vi "Get_Variant_Cluster_Element_Names.vi"(8 "error in (no error)":errorcluster, 11 "Cluster in":variant) -> (0 "error out":errorcluster, 2 "Element names":string[](array[string]), 3 "Cluster out":variant)   [LabVIEW 2012]
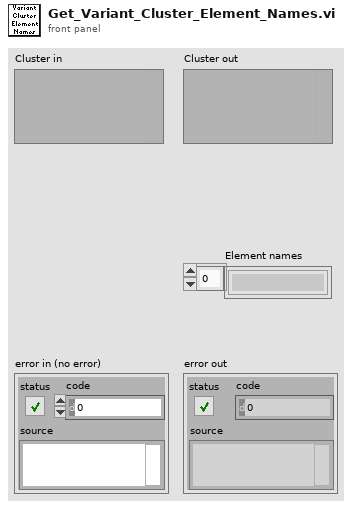
[diagram p1: front panel]
types:
  T1 = cluster{"length":u16, "private":u8, "type":enum8{"<Null>", "I8", "I16", "I32", "I64", "U8", "U16", "U32", "U64", "SGL", "DBL", "EXT", "CSG", "CDB", "CXT", "0x0F", "0x10", "0x11", "0x12", "0x13", "0x14", "Enum U8", "Enum U16", "Enum U32", "Enum U64", "SGL PQ", "DBL PQ", "EXT PQ", "CSG PQ", "CDB PQ", "CXT PQ", "0x1F", "0x20", "Boolean", "0x22", "0x23", "0x24", "0x25", "0x26", "0x27", "0x28", "0x29", "0x2A", "0x2B", "0x2C", "0x2D", "0x2E", "0x2F", "String", "0x31", "Path", "Pict", "0x34", "0x35", "0x36", "DAQ", "0x38", "0x39", "0x3A", "0x3B", "0x3C", "0x3D", "0x3E", "0x3F", "Array", "0x41", "0x42", "0x43", "0x44", "0x45", "0x46", "0x47", "0x48", "0x49", "0x4A", "0x4B", "0x4C", "0x4D", "0x4E", "0x4F", "Cluster", "0x51", "0x52", "Variant", "Waveform", "0x55", "0x56", "0x57", "0x58", "0x59", "0x5A", "0x5B", "0x5C", "0x5D", "0x5E", "0x5F", "0x60", "0x61", "0x62", "0x63", "0x64", "0x65", "0x66", "0x67", "0x68", "0x69", "0x6A", "0x6B", "0x6C", "0x6D", "0x6E", "0x6F", "Refnum"}, "# elements":u16}
  T2 = enum8{"<Null>", "I8", "I16", "I32", "I64", "U8", "U16", "U32", "U64", "SGL", "DBL", "EXT", "CSG", "CDB", "CXT", "0x0F", "0x10", "0x11", "0x12", "0x13", "0x14", "Enum U8", "Enum U16", "Enum U32", "Enum U64", "SGL PQ", "DBL PQ", "EXT PQ", "CSG PQ", "CDB PQ", "CXT PQ", "0x1F", "0x20", "Boolean", "0x22", "0x23", "0x24", "0x25", "0x26", "0x27", "0x28", "0x29", "0x2A", "0x2B", "0x2C", "0x2D", "0x2E", "0x2F", "String", "0x31", "Path", "Pict", "0x34", "0x35", "0x36", "DAQ", "0x38", "0x39", "0x3A", "0x3B", "0x3C", "0x3D", "0x3E", "0x3F", "Array", "0x41", "0x42", "0x43", "0x44", "0x45", "0x46", "0x47", "0x48", "0x49", "0x4A", "0x4B", "0x4C", "0x4D", "0x4E", "0x4F", "Cluster", "0x51", "0x52", "Variant", "Waveform", "0x55", "0x56", "0x57", "0x58", "0x59", "0x5A", "0x5B", "0x5C", "0x5D", "0x5E", "0x5F", "0x60", "0x61", "0x62", "0x63", "0x64", "0x65", "0x66", "0x67", "0x68", "0x69", "0x6A", "0x6B", "0x6C", "0x6D", "0x6E", "0x6F", "Refnum"}
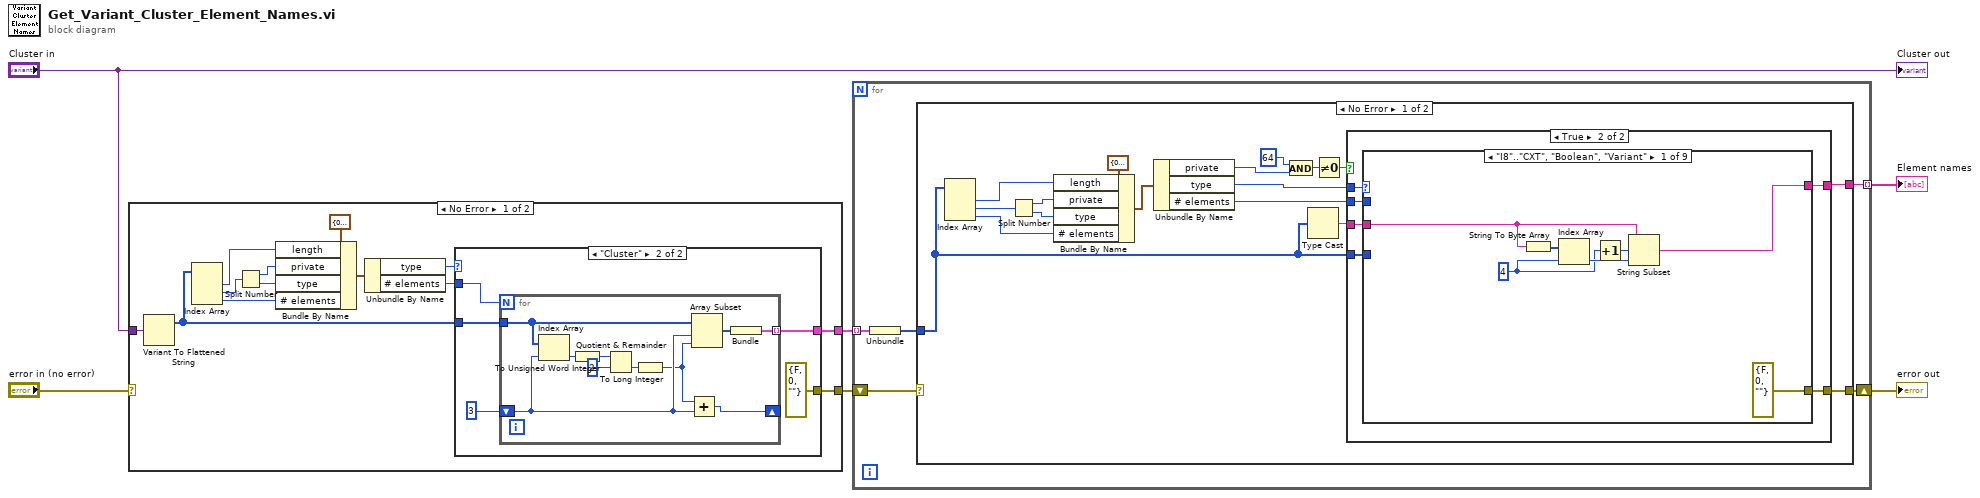
[diagram p0: block diagram]
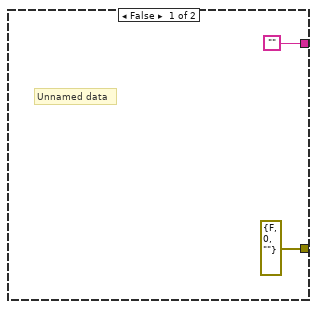
[diagram p2: hidden frame]
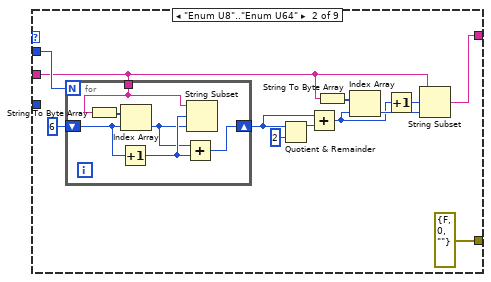
[diagram p3: hidden frame]
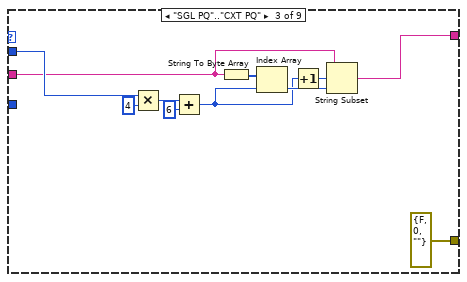
[diagram p4: hidden frame]
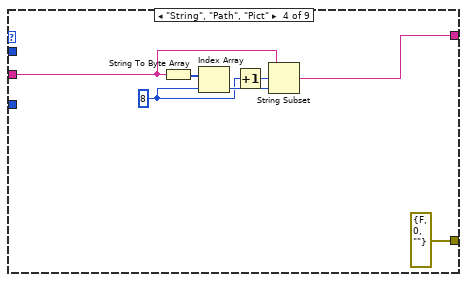
[diagram p5: hidden frame]
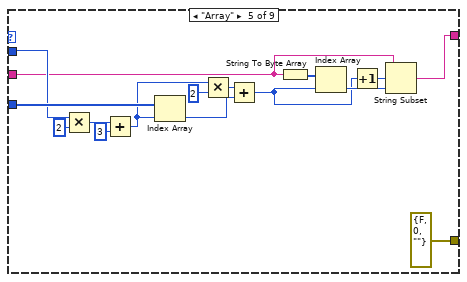
[diagram p6: hidden frame]
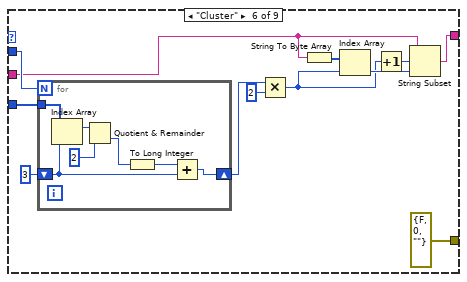
[diagram p7: hidden frame]
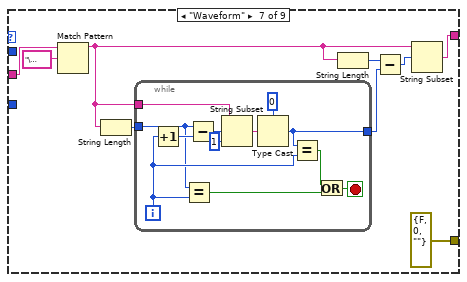
[diagram p8: hidden frame]
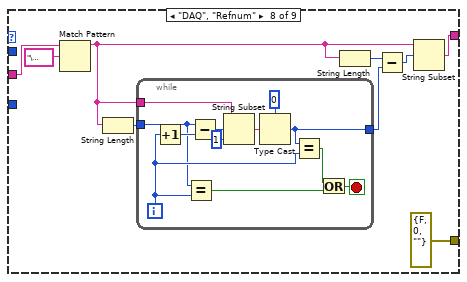
[diagram p9: hidden frame]
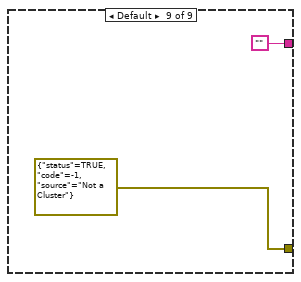
[diagram p10: hidden frame]
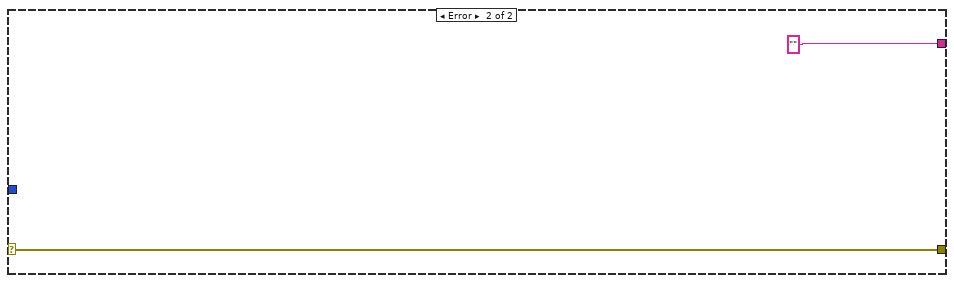
[diagram p11: hidden frame]
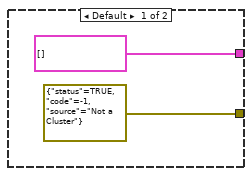
[diagram p12: hidden frame]
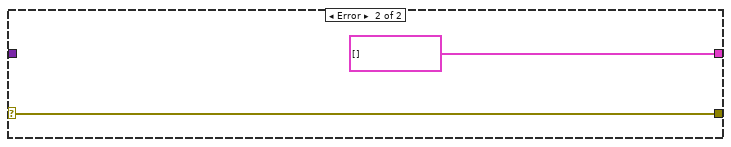
[diagram p13: hidden frame]
diagram:
  n1 = case shown="No Error" "error in (no error)" {
    selector: "error in (no error)" -> [_ w37]
    tunnel: [w17 cluster{i16[]}[] []] -> w4
    tunnel: [w16 w37] -> w3
    tunnel: "Cluster in" -> [w8 _]
    frame No Error {
      n2 = Variant To Flattened String(Variant=w8) -> (1:w7:i16[])  [unwired: 1 out]
      n3 = Index Array(array=w7) -> (element #1=w14:i16, element #2=w11:i16, element #3=w10:i16)  [unwired: 3 in]
      n4 = Split Number(x=w11) -> (hi(x)=w13:u8, lo(x)=w12:u8)
      n5 = Bundle By Name(cluster=T1 {"length"=0, "private"=0, "type"=enum."<Null>", "# elements"=0} ("Type Descriptor Header"), "length"=w14, "private"=w13, "type"=w12, "# elements"=w10) -> (w9:T1)
      n6 = Unbundle By Name(w9) -> ("type"=w19:T2, "# elements"=w18:u16)
      n7 = case shown="\"Cluster\"" w19 {
        tunnel: w18 -> [_ w25]
        tunnel: w7 -> [_ w24]
        tunnel: [cluster{i16[]}[] [] w23] -> w17
        tunnel: [errorcluster {"status"=TRUE, "code"=-1, "source"="Not a Cluster"} ("error out") errorcluster {"status"=FALSE, "code"=0, "source"=""} ("error out")] -> w16
        frame Default {
        }
        frame "Cluster" {
          n8 = for {
            N: w25 -> [_]
            shift-right: [w34] -> _
            shift-left: 3 -> [w33]
            tunnel: w24 -> [w35]
            tunnel: [w29] -> w23 mode=indexing
            n9 = Index Array(array=w35, index=w33) -> (element=w31:i16)
            n10 = To Unsigned Word Integer(number=w31) -> (unsigned 16bit integer=w28:u16)
            n11 = Quotient & Remainder(x=w28, y=u16 2) -> (floor(x/y)=w32:u16)  [unwired: 1 out]
            n12 = To Long Integer(number=w32) -> (32bit integer=w27:i32)
            n13 = Add(x=w27, y=w33) -> (x+y=w34:i32)
            n14 = Array Subset(array=w35, index=w33, length=w27) -> (w36:i16[])
            n15 = Bundle(w36) -> (w29:cluster{i16[]})  [unwired: 1 in]
          }
        }
      }
    }
    frame Error {
    }
  }
  n16 = for {
    tunnel: w4 -> [w42] mode=indexing
    shift-right: [w40] -> w2
    shift-left: w3 -> [w41]
    tunnel: [w39] -> w1 mode=indexing
    n17 = Unbundle(w42) -> (w43:i16[])
    n18 = case shown="No Error" w41 {
      selector: w41 -> [_ w192]
      tunnel: w43 -> [w45 _]
      tunnel: [w58 "" ("Last PString")] -> w39
      tunnel: [w52 w192] -> w40
      frame No Error {
        n19 = Index Array(array=w45) -> (element #1=w47:i16, element #2=w50:i16, element #3=w51:i16)  [unwired: 3 in]
        n20 = Split Number(x=w50) -> (hi(x)=w48:u8, lo(x)=w49:u8)
        n21 = Bundle By Name(cluster=T1 {"length"=0, "private"=0, "type"=enum."<Null>", "# elements"=0} ("Type Descriptor Header"), "length"=w47, "private"=w48, "type"=w49, "# elements"=w51) -> (w44:T1)
        n22 = Unbundle By Name(w44) -> ("private"=w54:u8, "type"=w53:T2, "# elements"=w60:u16)
        n23 = And(x=u8 64, y=w54) -> (x .and. y?=w57:u8)
        n24 = Type Cast(x=w45) -> (*(type *) &x=w59:string)  [unwired: 1 in]
        n25 = Not Equal To 0?(x=w57) -> (x != 0?=w56:bool)
        n26 = case shown="True" w56 {
          tunnel: [errorcluster {"status"=FALSE, "code"=0, "source"=""} ("error out") w68] -> w52
          tunnel: w53 -> [_ w67]
          tunnel: w59 -> [_ w66]
          tunnel: ["" w65] -> w58
          tunnel: w60 -> [_ w64]
          tunnel: w45 -> [_ w63]
          frame False {
            # "Unnamed data"
          }
          frame True {
            n27 = case shown="\"I8\"..\"CXT\", \"Boolean\", \"Variant\"" w67 {
              tunnel: [errorcluster {"status"=FALSE, "code"=0, "source"=""} ("error out") errorcluster {"status"=FALSE, "code"=0, "source"=""} ("error out") errorcluster {"status"=FALSE, "code"=0, "source"=""} ("error out") errorcluster {"status"=FALSE, "code"=0, "source"=""} ("error out") errorcluster {"status"=FALSE, "code"=0, "source"=""} ("error out") errorcluster {"status"=FALSE, "code"=0, "source"=""} ("error out") errorcluster {"status"=FALSE, "code"=0, "source"=""} ("error out") errorcluster {"status"=FALSE, "code"=0, "source"=""} ("error out") errorcluster {"status"=TRUE, "code"=-1, "source"="Not a Cluster"} ("error out")] -> w68
              tunnel: w66 -> [w69 w77 w95 w106 w113 w130 w148 w169 _]
              tunnel: [w70 w76 w94 w105 w112 w128 w147 w168 ""] -> w65
              tunnel: w64 -> [_ w84 w103 _ w119 w138 _ _ _]
              tunnel: w63 -> [_ _ _ _ w126 w137 _ _ _]
              frame "I8".."CXT", "Boolean", "Variant" {
                w71 = 4 ("offset (0)")
                n28 = String To Byte Array(string=w69) -> (unsigned byte array=w74:u8[])
                n29 = Index Array(array=w74, index=w71) -> (element=w72:u8)
                n30 = Increment(x=w71) -> (x+1=w73:i32)
                n31 = String Subset(string=w69, offset (0)=w73, length (rest)=w72) -> (substring=w70:string)
              }
              frame "Enum U8".."Enum U64" {
                n32 = for {
                  N: w84 -> [_]
                  tunnel: w77 -> [w90]
                  shift-right: [w89] -> w86
                  shift-left: 6 -> [w88]
                  n33 = String To Byte Array(string=w90) -> (unsigned byte array=w93:u8[])
                  n34 = Increment(x=w88) -> (x+1=w92:i32)
                  n35 = Index Array(array=w93, index=w88) -> (element=w91:u8)
                  n36 = Add(x=w91, y=w92) -> (x+y=w89:i32)
                  n37 = String Subset(string=w90, offset (0)=w92, length (rest)=w91) -> ()  [unwired: 1 out]
                }
                n38 = Quotient & Remainder(x=w86, y=2) -> (x-y*floor(x/y)=w82:i32)  [unwired: 1 out]
                n39 = Add(x=w86, y=w82) -> (x+y=w78:i32)
                n40 = String To Byte Array(string=w77) -> (unsigned byte array=w81:u8[])
                n41 = Index Array(array=w81, index=w78) -> (element=w79:u8)
                n42 = Increment(x=w78) -> (x+1=w80:i32)
                n43 = String Subset(string=w77, offset (0)=w80, length (rest)=w79) -> (substring=w76:string)
              }
              frame "SGL PQ".."CXT PQ" {
                n44 = Multiply(x=w103, y=u16 4) -> (x*y=w101:u16)
                n45 = Add(x=w101, y=u16 6) -> (x+y=w96:u16)
                n46 = String To Byte Array(string=w95) -> (unsigned byte array=w97:u8[])
                n47 = Index Array(array=w97, index=w96) -> (element=w99:u8)
                n48 = Increment(x=w96) -> (x+1=w98:u16)
                n49 = String Subset(string=w95, offset (0)=w98, length (rest)=w99) -> (substring=w94:string)
              }
              frame "String", "Path", "Pict" {
                w107 = 8 ("offset (0)")
                n50 = String To Byte Array(string=w106) -> (unsigned byte array=w108:u8[])
                n51 = Index Array(array=w108, index=w107) -> (element=w110:u8)
                n52 = Increment(x=w107) -> (x+1=w109:i32)
                n53 = String Subset(string=w106, offset (0)=w109, length (rest)=w110) -> (substring=w105:string)
              }
              frame "Array" {
                n54 = Multiply(x=w119, y=u16 2) -> (x*y=w121:u16)
                n55 = Add(x=w121, y=u16 3) -> (x+y=w118:u16)
                n56 = Index Array(array=w126, index=w118) -> (element=w123:i16)
                n57 = Multiply(x=w118, y=u16 2) -> (x*y=w124:u16)
                n58 = Add(x=w124, y=w123) -> (x+y=w114:u16)
                n59 = String To Byte Array(string=w113) -> (unsigned byte array=w117:u8[])
                n60 = Index Array(array=w117, index=w114) -> (element=w115:u8)
                n61 = Increment(x=w114) -> (x+1=w116:u16)
                n62 = String Subset(string=w113, offset (0)=w116, length (rest)=w115) -> (substring=w112:string)
              }
              frame "Cluster" {
                n63 = for {
                  N: w138 -> [_]
                  shift-right: [w145] -> w135
                  shift-left: 3 -> [w144]
                  tunnel: w137 -> [w146]
                  n64 = Index Array(array=w146, index=w144) -> (element=w142:i16)
                  n65 = Quotient & Remainder(x=w142, y=i16 2) -> (floor(x/y)=w143:i16)  [unwired: 1 out]
                  n66 = To Long Integer(number=w143) -> (32bit integer=w140:i32)
                  n67 = Add(x=w140, y=w144) -> (x+y=w145:i32)
                }
                n68 = Multiply(x=w135, y=2) -> (x*y=w129:i32)
                n69 = String To Byte Array(string=w130) -> (unsigned byte array=w131:u8[])
                n70 = Index Array(array=w131, index=w129) -> (element=w133:u8)
                n71 = Increment(x=w129) -> (x+1=w132:i32)
                n72 = String Subset(string=w130, offset (0)=w132, length (rest)=w133) -> (substring=w128:string)
              }
              frame "Waveform" {
                n73 = Match Pattern(string=w148, regular expression="\u0000$" ("*(type *) &x")) -> (before substring=w150:string)  [unwired: 1 in, 3 out]
                n74 = String Length(string=w150) -> (length=w149:i32)
                n75 = while {
                  tunnel: [w162] -> w154
                  tunnel: w149 -> [w157]
                  tunnel: w150 -> [w166]
                  i -> [w160]
                  stop <- w159 stop-if-true
                  n76 = Increment(x=w160) -> (x+1=w161:i32)
                  n77 = Equal?(x=w157, y=w160) -> (x = y?=w156:bool)
                  n78 = Subtract(x=w157, y=w161) -> (x-y=w165:i32)
                  n79 = String Subset(string=w166, offset (0)=w165, length (rest)=1 ("length (rest)")) -> (substring=w164:string)
                  n80 = Type Cast(type=u8 0, x=w164) -> (*(type *) &x=w162:u8)
                  n81 = Equal?(x=w162, y=w160) -> (x = y?=w158:bool)
                  n82 = Or(x=w158, y=w156) -> (x .or. y?=w159:bool)
                }
                n83 = String Length(string=w150) -> (length=w152:i32)
                n84 = Subtract(x=w152, y=w154) -> (x-y=w153:i32)
                n85 = String Subset(string=w150, offset (0)=w153) -> (substring=w147:string)  [unwired: 1 in]
              }
              frame "DAQ", "Refnum" {
                n86 = Match Pattern(string=w169, regular expression="\u0000$" ("*(type *) &x")) -> (before substring=w174:string)  [unwired: 1 in, 3 out]
                n87 = String Length(string=w174) -> (length=w175:i32)
                n88 = while {
                  tunnel: [w183] -> w170
                  tunnel: w175 -> [w178]
                  tunnel: w174 -> [w187]
                  i -> [w181]
                  stop <- w180 stop-if-true
                  n89 = Increment(x=w181) -> (x+1=w182:i32)
                  n90 = Equal?(x=w178, y=w181) -> (x = y?=w177:bool)
                  n91 = Subtract(x=w178, y=w182) -> (x-y=w186:i32)
                  n92 = String Subset(string=w187, offset (0)=w186, length (rest)=1 ("length (rest)")) -> (substring=w185:string)
                  n93 = Type Cast(type=u8 0, x=w185) -> (*(type *) &x=w183:u8)
                  n94 = Equal?(x=w183, y=w181) -> (x = y?=w179:bool)
                  n95 = Or(x=w179, y=w177) -> (x .or. y?=w180:bool)
                }
                n96 = String Length(string=w174) -> (length=w172:i32)
                n97 = Subtract(x=w172, y=w170) -> (x-y=w171:i32)
                n98 = String Subset(string=w174, offset (0)=w171) -> (substring=w168:string)  [unwired: 1 in]
              }
              frame Default {
              }
            }
          }
        }
      }
      frame Error {
      }
    }
  }
  "error out" <- w2
  "Element names" <- w1
  "Cluster out" <- "Cluster in"
